vi "Crop_dss.vi"(5 "Field_Astrom":T1 {"CRVAL" format="%.6g"; "CD" format="%_7g"}, 7 "Img Astrometry":T1, 8 "Y Scale.Range":T2, 9 "X Scale.Range":T2, 10 "Img DEC":dbl, 11 "Img RA":dbl) -> (0 "lpixel (-1,-1: rest)":cluster{"X":i32, "Y":i32}={"X"=-1, "Y"=-1}, 1 "fpixel (1,1)":cluster{"X":i32, "Y":i32}={"X"=1, "Y"=1})   [LabVIEW 2019]
uses:
  <vilib>/Utility/miscctls.llb/LVRangeTypeDef.ctl
panel:
  out "Y":dbl[](array[numeric])
  out "X":dbl[](array[numeric])
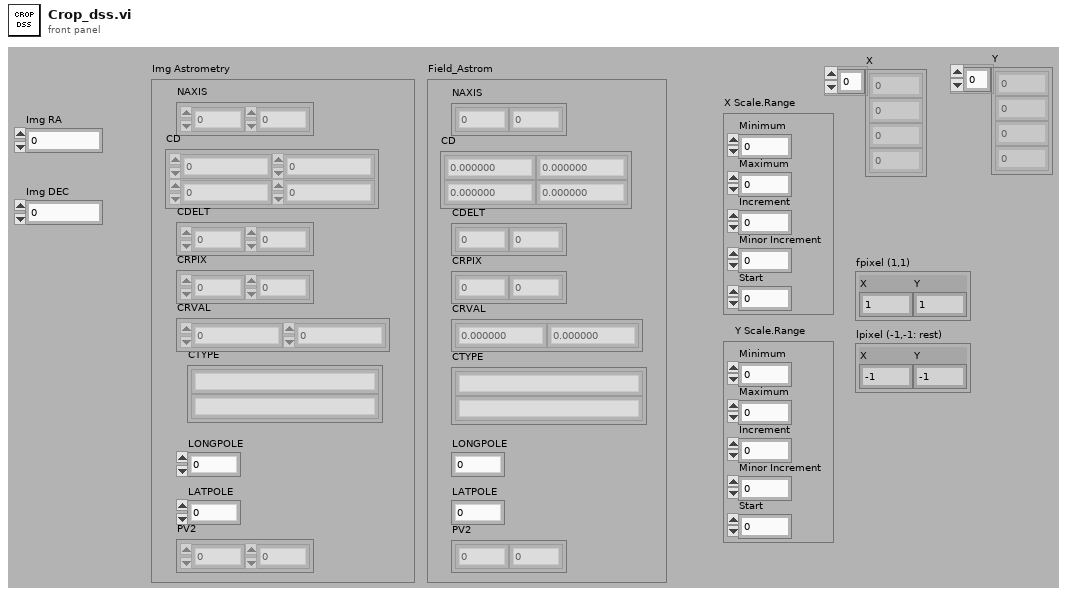
[diagram p1: front panel]
types:
  T1 = cluster{"NAXIS":dbl[], "CD":dbl[][], "CDELT":dbl[], "CRPIX":dbl[], "CTYPE":string[], "CRVAL":dbl[], "LONGPOLE":dbl, "LATPOLE":dbl, "PV2":dbl[]}
  T2 = typedef "LVRangeTypeDef.ctl" = cluster{"Minimum":dbl, "Maximum":dbl, "Increment":dbl, "Minor Increment":dbl, "Start":dbl}
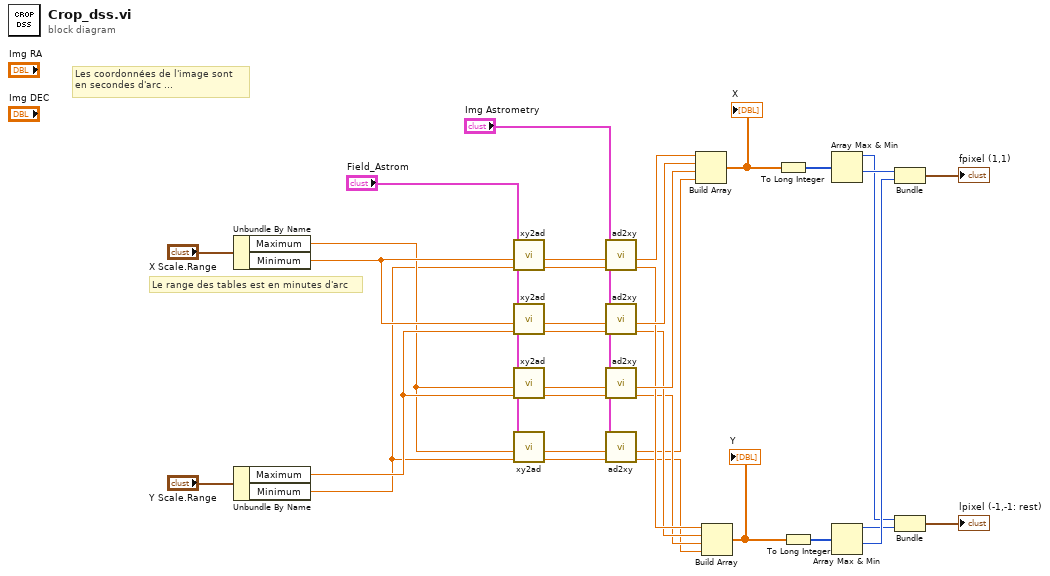
[diagram p0: block diagram]
diagram:
  # "Les coordonnées de l'image sont\nen secondes d'arc ..."
  # "Le range des tables est en minutes d'arc"
  n1 = Unbundle By Name("X Scale.Range") -> ("Maximum"=w3:dbl, "Minimum"=w5:dbl)
  n2 = Unbundle By Name("Y Scale.Range") -> ("Maximum"=w4:dbl, "Minimum"=w2:dbl)
  n3 = call "xy2ad.vi"("Y (px)"=w2, "X (px)"=w5, "Astrometry"="Field_Astrom") -> ("DEC (°)"=w12:dbl, "RA (°)"=w13:dbl)  [unwired: 5 in, 2 out]
  n4 = call "xy2ad.vi"("Y (px)"=w4, "X (px)"=w5, "Astrometry"="Field_Astrom") -> ("DEC (°)"=w10:dbl, "RA (°)"=w11:dbl)  [unwired: 5 in, 2 out]
  n5 = call "xy2ad.vi"("Y (px)"=w4, "X (px)"=w3, "Astrometry"="Field_Astrom") -> ("DEC (°)"=w8:dbl, "RA (°)"=w9:dbl)  [unwired: 5 in, 2 out]
  n6 = call "xy2ad.vi"("Y (px)"=w2, "X (px)"=w3, "Astrometry"="Field_Astrom") -> ("DEC (°)"=w6:dbl, "RA (°)"=w7:dbl)  [unwired: 5 in, 2 out]
  n7 = call "ad2xy.vi"("DEC"=w12, "RA"=w13, "Astrometry"="Img Astrometry") -> ("Y"=w28:dbl, "X"=w31:dbl)  [unwired: 6 in, 1 out]
  n8 = call "ad2xy.vi"("DEC"=w10, "RA"=w11, "Astrometry"="Img Astrometry") -> ("Y"=w27:dbl, "X"=w30:dbl)  [unwired: 6 in, 1 out]
  n9 = call "ad2xy.vi"("DEC"=w8, "RA"=w9, "Astrometry"="Img Astrometry") -> ("Y"=w26:dbl, "X"=w29:dbl)  [unwired: 6 in, 1 out]
  n10 = call "ad2xy.vi"("DEC"=w6, "RA"=w7, "Astrometry"="Img Astrometry") -> ("Y"=w24:dbl, "X"=w25:dbl)  [unwired: 6 in, 1 out]
  n11 = Build Array(w31, w30, w29, w25) -> (w23:dbl[])
  "X" <- w23
  n12 = Build Array(w28, w27, w26, w24) -> (w14:dbl[])
  "Y" <- w14
  n13 = To Long Integer(number=w23) -> (32bit integer=w16:i32[])
  n14 = To Long Integer(number=w14) -> (32bit integer=w15:i32[])
  n15 = Array Max & Min(array=w16) -> (max value=w17:i32, min value=w21:i32)  [unwired: 2 out]
  n16 = Array Max & Min(array=w15) -> (max value=w18:i32, min value=w20:i32)  [unwired: 2 out]
  n17 = Bundle(w21, w20) -> (→"fpixel (1,1)":cluster{i32, i32})  [unwired: 1 in]
  n18 = Bundle(w17, w18) -> (→"lpixel (-1,-1: rest)":cluster{i32, i32})  [unwired: 1 in]
